vi "MDAQ_CursorHelp.vi"(9 "Input Cluster":T1 {"GATESTOP" format="%04x"; "GATESTRT" format="%04x"; "AMPLITUDE" format="%04x"; "M_CYCLES" format="%04x"; "N_CYCLES" format="%04x"; "STEP" format="%04x"; "BASE" format="%04x"; "CHAN" format="%04x"}) -> (1 "X-Cursor-1":dbl, 2 "X-Cursor-0":dbl)   [LabVIEW 2021]
uses:
  Status_Cluster.ctl
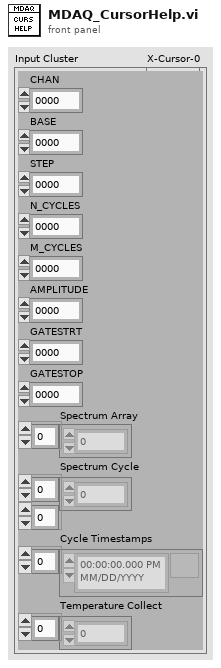
[diagram p1: front panel]
types:
  T1 = typedef "Status_Cluster.ctl" = cluster{"CHAN":u32, "BASE":u32, "STEP":u32, "N_CYCLES":u32, "M_CYCLES":u32, "AMPLITUDE":u32, "GATESTRT":u32, "GATESTOP":u32, "Spectrum Array":u32[], "Spectrum Cycle":u32[][], "Cycle Timestamps":timestamp[], "Temperature Collect":dbl[]}
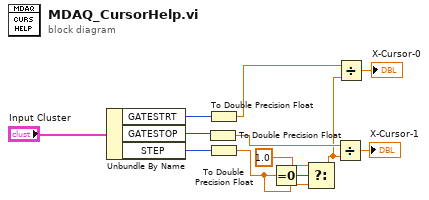
[diagram p0: block diagram]
diagram:
  n1 = Unbundle By Name("Input Cluster") -> ("GATESTRT"=w6:u32, "GATESTOP"=w10:u32, "STEP"=w8:u32)
  n2 = To Double Precision Float(number=w10) -> (double precision float=w9:dbl)
  n3 = To Double Precision Float(number=w6) -> (double precision float=w1:dbl)
  n4 = To Double Precision Float(number=w8) -> (double precision float=w5:dbl)
  n5 = Equal To 0?(x=w5) -> (x = 0?=w7:bool)
  n6 = Select(t=1.0, s=w7, f=w5) -> (s? t:f=w2:dbl)
  n7 = Divide(x=w9, y=w2) -> (x/y=→"X-Cursor-1":dbl)
  n8 = Divide(x=w1, y=w2) -> (x/y=→"X-Cursor-0":dbl)
